vi "GetSensorBdcstEvents.vi"(7 "error in (no error)":errorcluster) -> (3 "Event Registration Refnum":refnum<event-registration>, 5 "error out":errorcluster)   [LabVIEW 2018, in "Test.lvclass"]
uses:
  Test.lvclass
  Sensor/SensorShared/clEventType.ctl
  Sensor/SensorShared/SensorShared.lvlib
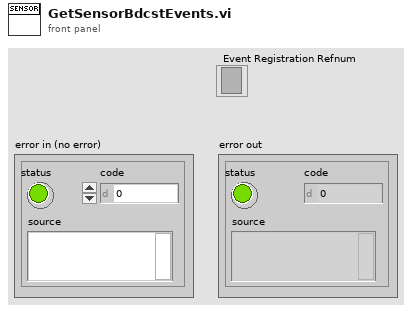
[diagram p1: front panel]
types:
  T1 = typedef "SensorShared.lvlib/clBroadcastEvents.ctl" = cluster{"DidInit":refnum<user-event>, "StatusUpdate":refnum<user-event>, "ErrorReport":refnum<user-event>, "DidStop":refnum<user-event>, "PathToINI":refnum<user-event>, "SensorReport":refnum<user-event>, "SensorConfig":refnum<user-event>}
  T2 = cluster{"SensorConfig":refnum<user-event>, "ErrorReport":refnum<user-event>, "SensorReport":refnum<user-event>}
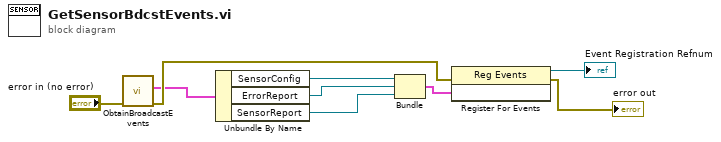
[diagram p0: block diagram]
diagram:
  n1 = call "ObtainBroadcastEvents.vi"("error in (no error)"="error in (no error)") -> ("error out"=w4:errorcluster, "clBroadcastEvents"=w3:T1)  [unwired: 9 in]
  n2 = Unbundle By Name(w3) -> ("SensorConfig"=w9:refnum<user-event>, "ErrorReport"=w7:refnum<user-event>, "SensorReport"=w2:refnum<user-event>)
  n3 = Bundle("SensorConfig"=w9, "ErrorReport"=w7, "SensorReport"=w2) -> (w8:T2)  [unwired: 1 in]
  n4 = register-events(error in=w4, w8) -> (reference out=→"Event Registration Refnum":refnum<event-registration>, error out=→"error out":errorcluster)  [unwired: 1 in]
